vi "Initialize.vi"(8 "error in (no error)":errorcluster, 11 "handler in":refnum<class "Handler.lvclass">) -> (0 "error out":errorcluster, 3 "handler out":refnum<class "Handler.lvclass">)   [LabVIEW 2024, in "Logging.lvlib" / "Handler.lvclass"]
uses:
  Handler.lvclass
  Handler.lvclass/Handler.ctl
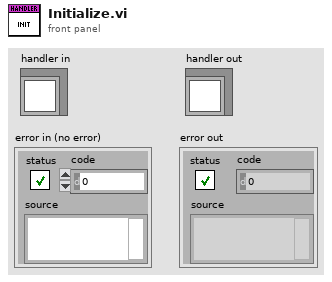
[diagram p1: front panel]
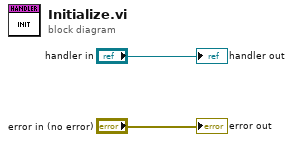
[diagram p0: block diagram]
diagram:
  "error out" <- "error in (no error)"
  "handler out" <- "handler in"
